vi "Get Section Name.vi"(8 "Error In":errorcluster, 10 "Object name":string, 11 "object":refnum<class>) -> (0 "Error Out":errorcluster, 2 "Section out":string)   [LabVIEW 2015]
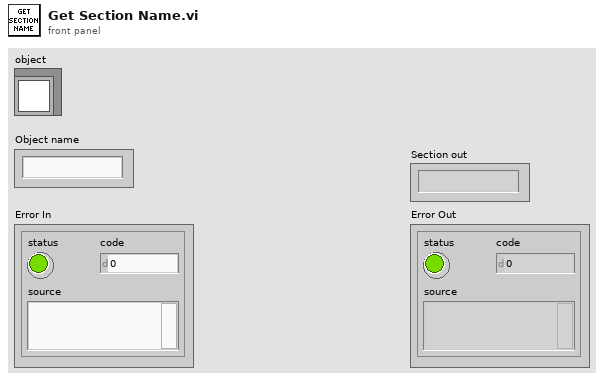
[diagram p1: front panel]
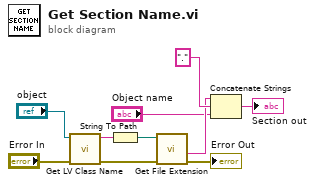
[diagram p0: block diagram]
diagram:
  n1 = call <vilib>:"Get LV Class Name.vi"("error in (no error)"="Error In", "object"="object") -> ("error out"=w7:errorcluster, "class name"=w9:string)  [unwired: 8 in]
  n2 = String To Path(string=w9) -> (path=w5:path)
  n3 = call <vilib>:"Get File Extension.vi"("error in (no error)"=w7, "file"=w5) -> ("error out"=→"Error Out":errorcluster, "filename without extension"=w6:string)  [unwired: 5 in, 3 out]
  n4 = Concatenate Strings(w6, "." ("string"), "Object name") -> (→"Section out":string)
